vi "Synchronization Mode.vi"() -> ()   [LabVIEW 2018]
uses:
  <resource>/objmgr/IndComECAT.rc
panel:
  out "Array":u8[](array[numeric])
  in  "Decimal Input":i32
  out "String":string
  out "Abort Code":u32
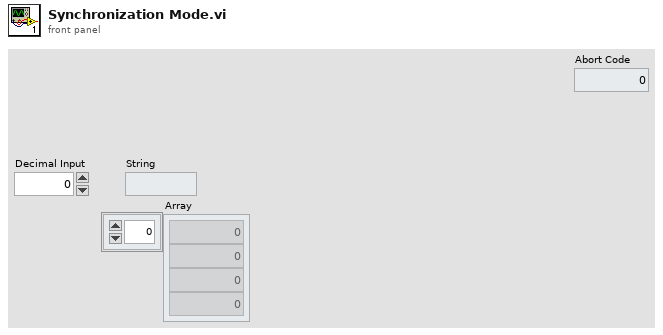
[diagram p1: front panel]
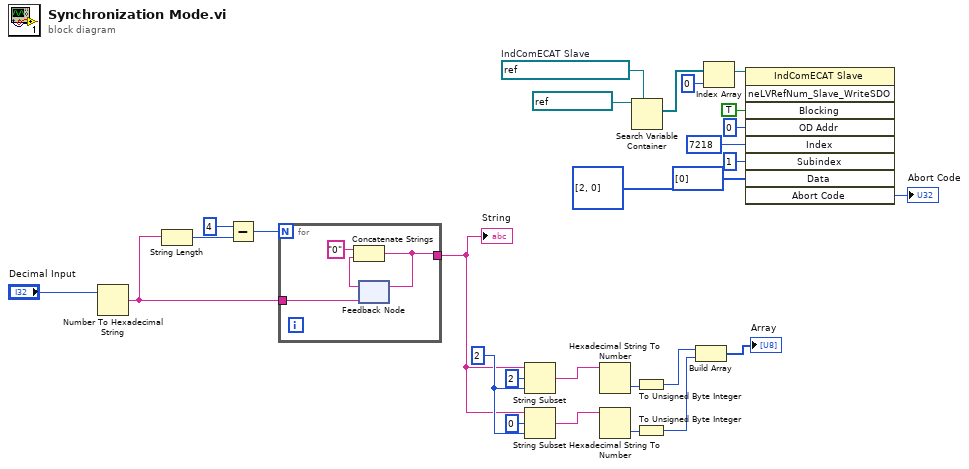
[diagram p0: block diagram]
diagram:
  (unwired) u8[] [0] ("Data")
  w5 = refnum<k21> refnum  # IndComECAT Slave
  w20 = 2 ("length (rest)")
  n1 = Number To Hexadecimal String(2:"Decimal Input") -> (0:w13:string)  [unwired: 1 in]
  n2 = String Length(string=w13) -> (length=w14:i32)
  n3 = Subtract(x=4, y=w14) -> (x-y=w15:i32)
  n4 = for {
    N: w15 -> [_]
    tunnel: w13 -> [w29]
    tunnel: [w28] -> w19
    n5 = feedback #1(w29) -> (w30:string)
    n6 = Concatenate Strings("0" ("string"), w30) -> (w28:string)
    n7 = feedback-in #1(w28) -> ()
  }
  "String" <- w19
  n8 = String Subset(string=w19, offset (0)=2, length (rest)=w20) -> (substring=w21:string)
  n9 = String Subset(string=w19, offset (0)=0, length (rest)=w20) -> (substring=w22:string)
  n10 = Hexadecimal String To Number(string=w21) -> (number=w23:u32)  [unwired: 2 in, 1 out]
  n11 = Hexadecimal String To Number(string=w22) -> (number=w24:u32)  [unwired: 2 in, 1 out]
  n12 = Search Variable Container(7:w5, 11:refnum<k21> "ni.var.io:/" ("container refnum in")) -> (2:w7:refnum<k21>[])  [unwired: 4 in, 2 out]
  n13 = To Unsigned Byte Integer(number=w23) -> (unsigned 8bit integer=w25:u8)
  n14 = To Unsigned Byte Integer(number=w24) -> (unsigned 8bit integer=w26:u8)
  n15 = Build Array(w25, w26) -> (→"Array":u8[])
  n16 = Index Array(array=w7, index=0) -> (element=w6:refnum<k21>)
  n17 = invoke class="IndComECAT Slave" method="neLVRefNum_Slave_WriteSDO"(reference=w6, "Blocking"=TRUE, "OD Addr"=u16 0, "Index"=u16 7218, "Subindex"=u8 1, "Data"=u8[] [2, 0]) -> ("Abort Code"=→"Abort Code":u32)  [unwired: 3 in, 8 out]
